vi "MD4Logger.Async.vi"(10 "Parameters":variant, 11 "Process":refnum<class "Process.lvclass">) -> ()   [LabVIEW 2019, in "MD4Logger Engine.lvlib"]
uses:
  MD4Logger Engine.lvlib
  <vilib>/NI/NIVS Inline Async API/_VS Inline Async API/Process/Process.lvclass
  Shared/Compiled.Settings.ctl
  <vilib>/NI/NIVS Inline Async API/_VS Inline Async API/Process/Process.lvclass/Process.ctl
  <vilib>/NI/NIVS Inline Async API/_Data Access Engine/Access Type Classes/Read/Read.lvclass/Read.ctl
  <vilib>/NI/NIVS Inline Async API/_Data Access Engine/Access Type Classes/Write/Write.lvclass/Write.ctl
  <vilib>/NI/NIVS Inline Async API/_Data Access Engine/Data Access Engine/Methods/Read.Data.vi
  <vilib>/NI/NIVS Inline Async API/_Data Access Engine/Data Access Engine/Methods/Write.Data.vi
  <vilib>/NI/NIVS Inline Async API/_VS Inline Async API/Process/Data Member Access/Read Data Access.vi
  <vilib>/NI/NIVS Inline Async API/_VS Inline Async API/Error Handling Process/SubVIs/Error.ConvertArray.vi
  <vilib>/NI/NIVS Inline Async API/_Data Access Engine/Access Type Classes/Read/Read.ProcessData.vi
  <vilib>/NI/NIVS Inline Async API/_Data Access Engine/Access Type Classes/Write/Write.ProcessData.vi
  <vilib>/NI/NIVS Inline Async API/_Data Access Engine/Data Access Engine/Methods/Write.Lookup.vi
  <vilib>/NI/NIVS Inline Async API/_Data Access Engine/Data Access Engine/Methods/Read.Lookup.vi
  <vilib>/NI/NIVS Inline Async API/_Data Access Engine/Data Access Engine/Data Access Engine.lvclass
  Shared/MD4Logger Shared.lvlib
  <vilib>/NI VeriStand/Custom Device Tools/Custom Device Utility Library/Custom Device Utility Library.lvlib
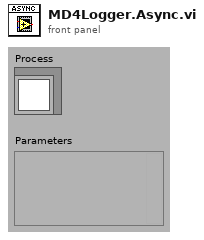
[diagram p1: front panel]
types:
  T1 = typedef "MD4Logger Shared.lvlib/Compiled.Settings.ctl" = cluster{"Name":string, "Folder Path":path, "Channnel Names":cluster{"Name":string, "Unit":string}[]}
  T2 = cluster{"Comment":string, "Time Source":string, "Author":string, "Department":string, "Project":string, "Subject":string}
  T3 = cluster{"History":string, "ID":string, "Vendor":string, "Version":string}
  T4 = typedef "Data Access Engine.lvlib/Data Access Engine.lvclass/Write.DVR.ctl" = refnum<data-value>
  T5 = typedef "Data Access Engine.lvlib/Data Access Engine.lvclass/Read.DVR.ctl" = refnum<data-value>
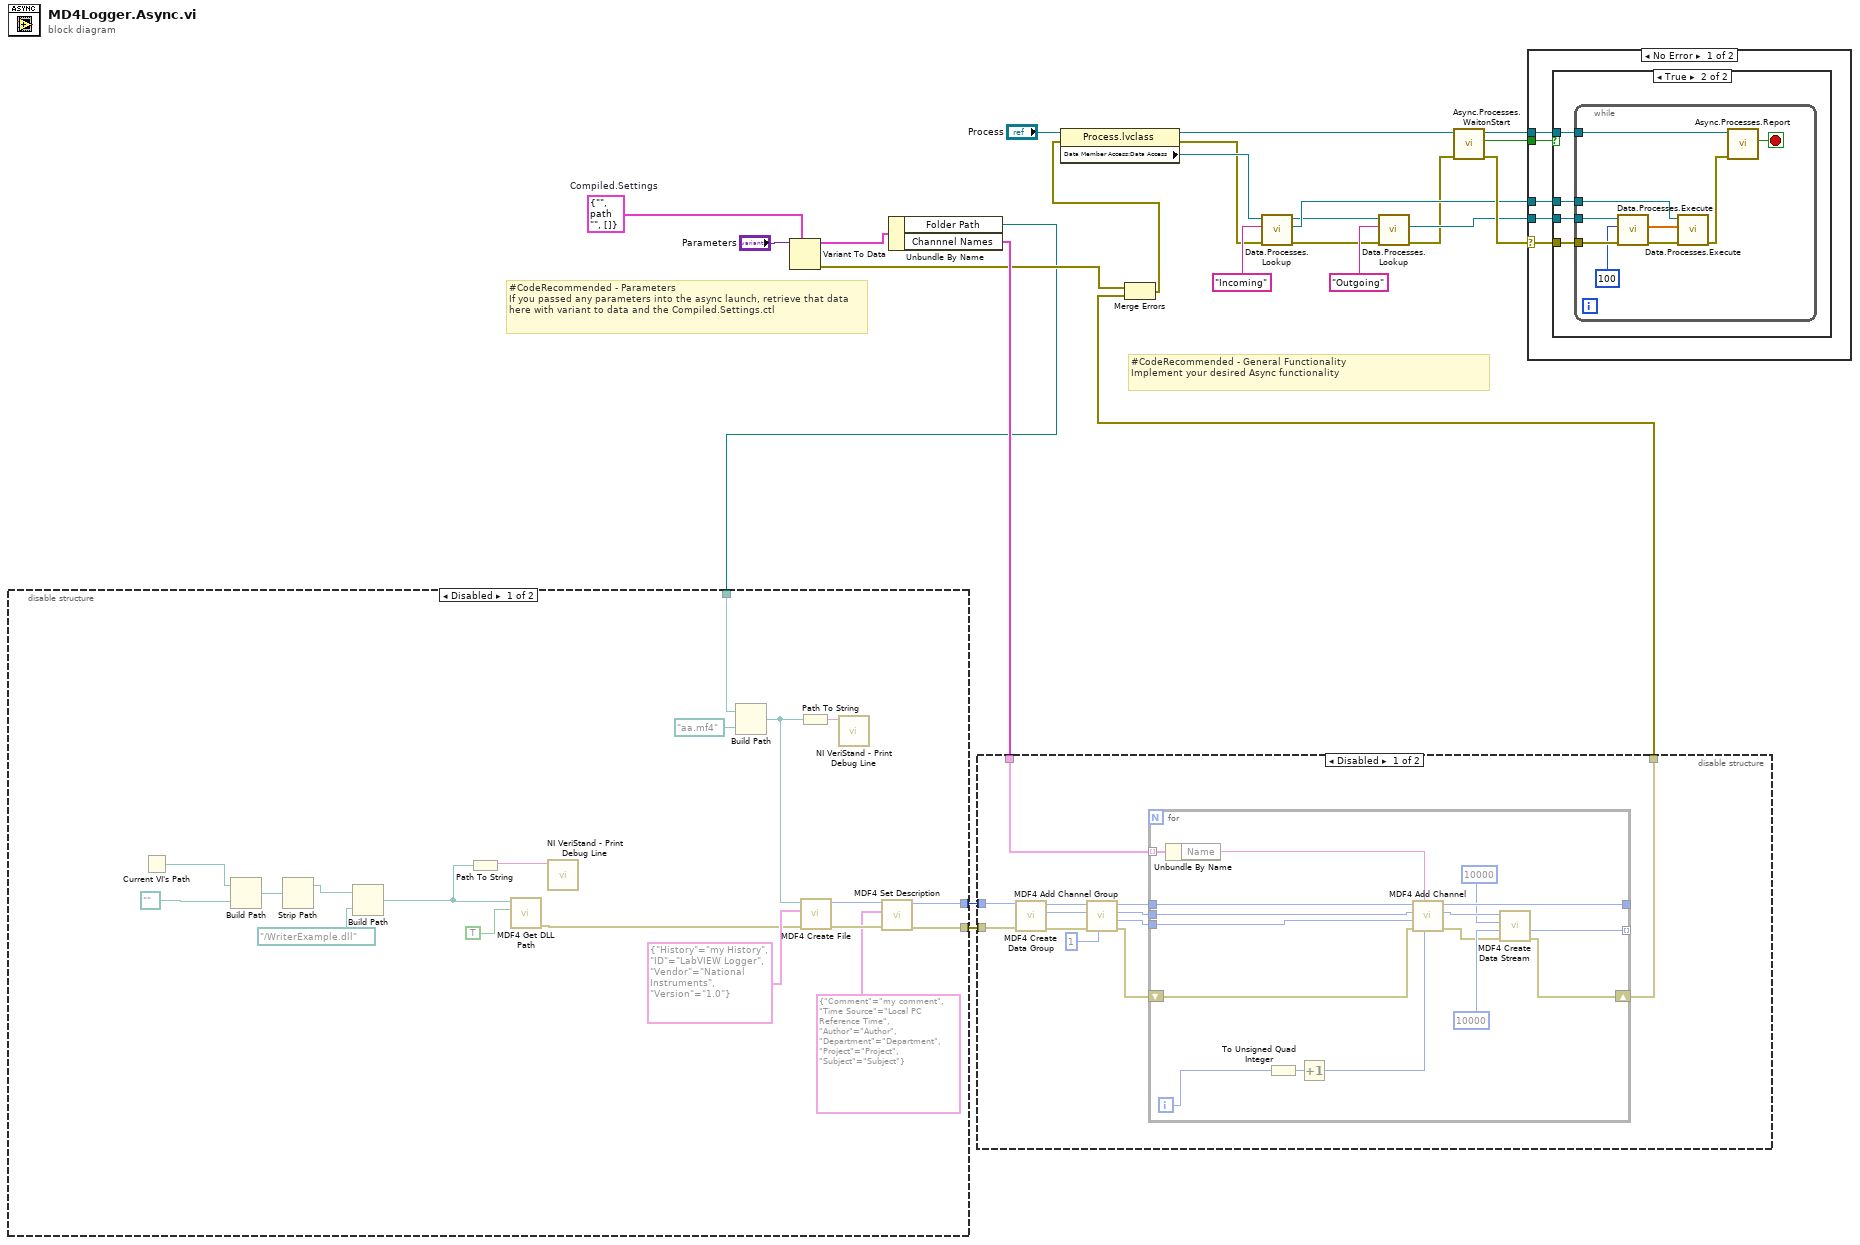
[diagram p0: block diagram]
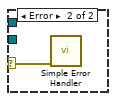
[diagram p5: hidden frame]
diagram:
  w9 = T1 {"Name"="", "Folder Path"=path "", "Channnel Names"=[]}  # Compiled.Settings
  # "#CodeRecommended - General Functionality\nImplement your desired Async functionality"
  # "#CodeRecommended - Parameters\nIf you passed any parameters into the async launch, retrieve that data here with variant to data and the Compiled.Settings.ctl"
  n1 = Variant To Data(type=w9, Variant="Parameters") -> (data=w8:T1, error out=w6:errorcluster)  [unwired: 1 in]
  n2 = Unbundle By Name(w8) -> ("Folder Path"=w1:path, "Channnel Names"=w7:cluster{"Name":string, "Unit":string}[])
  n3 = disable-structure shown="Disabled" {
    disable-tunnel: [w35 _] -> w3
    disable-tunnel: [w34 _] -> w2
    disable-tunnel: w1 -> [w26 _]
    frame Disabled {
      n4 = Current VI's Path() -> (path=w42:path)
      n5 = Build Path(base path=w42, name or relative path=path "..") -> (appended path=w40:path)
      n6 = Strip Path(path=w40) -> (stripped path=w39:path)  [unwired: 1 out]
      n7 = Build Path(base path=w39, name or relative path=path "../WriterExample.dll") -> (appended path=w29:path)
      n8 = Path To String(path=w29) -> (string=w43:string)
      n9 = call "MDF4 Get DLL Path.vi"("Init"=TRUE, "DLL Path"=w29) -> ("error out"=w30:errorcluster)  [unwired: 8 in, 1 out]
      n10 = call <vilib>:"NI VeriStand - Print Debug Line.vi"("Message"=w43) -> ()  [unwired: 10 in, 1 out]
      n11 = Build Path(base path=w26, name or relative path=path "aa.mf4") -> (appended path=w25:path)
      n12 = Path To String(path=w25) -> (string=w28:string)
      n13 = call "MDF4 Create File.vi"("Error In"=w30, "History"=T3 {"History"="my History", "ID"="LabVIEW Logger", "Vendor"="National Instruments", "Version"="1.0"}, "MDF4 File Path"=w25) -> ("Error Out"=w36:errorcluster, "MDF4 File Reference out"=w37:i64)  [unwired: 6 in]
      n14 = call <vilib>:"NI VeriStand - Print Debug Line.vi"("Message"=w28) -> ()  [unwired: 10 in, 1 out]
      n15 = call "MDF4 Set Description.vi"("Error In"=w36, "Comment"=T2 {"Comment"="my comment", "Time Source"="Local PC Reference Time", "Author"="Author", "Department"="Department", "Project"="Project", "Subject"="Subject"}, "MDF4 File Reference in"=w37) -> ("Error Out"=w35:errorcluster, "MDF4 File Reference out"=w34:i64)  [unwired: 7 in]
    }
    frame Enabled {
    }
  }
  n16 = disable-structure shown="Disabled" {
    disable-tunnel: w7 -> [w55 _]
    disable-tunnel: [w54 w72] -> w5
    disable-tunnel: w3 -> [w53 w72]
    disable-tunnel: w2 -> [w52 _]
    frame Disabled {
      n17 = call "MDF4 Create Data Group.vi"("Error In"=w53, "MDF4 File Reference in"=w52) -> ("Error Out"=w51:errorcluster, "Data Group Reference out"=w50:i64, "MDF4 File Reference out"=w49:i64)  [unwired: 7 in]
      n18 = call "MDF4 Add Channel Group.vi"("Record ID"=u64 1, "Error In"=w51, "Data Group Reference in"=w50, "MDF4 File Reference in"=w49) -> ("Error Out"=w48:errorcluster, "Channel Group Reference out"=w45:i64, "Data Group Reference out"=w46:i64, "MDF4 File Reference out"=w47:i64)  [unwired: 4 in]
      n19 = for {
        tunnel: [w71] -> _ mode=indexing
        tunnel: [w70] -> _
        shift-right: [w69] -> w54
        shift-left: w48 -> [w62]
        tunnel: w47 -> [w61]
        tunnel: w46 -> [w60]
        tunnel: w45 -> [w59]
        tunnel: w55 -> [w57] mode=indexing
        i -> [w63]
        n20 = Unbundle By Name(w57) -> ("Name"=w56:string)
        n21 = To Unsigned Quad Integer(1:w63) -> (0:w68:u64)
        n22 = Increment(x=w68) -> (x+1=w58:u64)
        n23 = call "MDF4 Add Channel.vi"("Channel ID"=w58, "Channel Name"=w56, "Error In"=w62, "Channel Group Reference in"=w59, "Data Group Reference in"=w60, "MDF4 File Reference in"=w61) -> ("Error Out"=w64:errorcluster, "Data Group Reference out"=w67:i64, "MDF4 File Reference out"=w70:i64)  [unwired: 3 in]
        n24 = call "MDF4 Create Data Stream.vi"("Error In"=w64, "Number of Samples per Read"=u32 10000, "Iterations"=u32 10000, "Data Group Reference in"=w67) -> ("Error Out"=w69:errorcluster, "Stream Reference out"=w71:i64)  [unwired: 5 in, 1 out]
      }
    }
    frame Enabled {
    }
  }
  n25 = Merge Errors(w6, w5) -> (w4:errorcluster)
  n26 = property class="Process.lvclass"(reference="Process", error in=w4) -> (reference out=w13:refnum<class "Process.lvclass">, error out=w11:errorcluster, "Data Member Access:Data Access"=w12:refnum<class "Data Access Engine.lvclass">)
  n27 = call-poly <vilib>:"Data.Processes.Lookup.vi"("error in (no error)"=w11, "Name"="Incoming", "Data Access API in"=w12) -> ("error out"=w18:errorcluster, "Ref"=w17:T4, "Data Access API out"=w16:refnum<class "Data Access Engine.lvclass">)  [unwired: 5 in, 1 out]
  n28 = call-poly <vilib>:"Data.Processes.Lookup.vi"("error in (no error)"=w18, "Name"="Outgoing", "Data Access API in"=w16) -> ("error out"=w15:errorcluster, "Ref"=w20:T5)  [unwired: 5 in, 2 out]
  n29 = call <vilib>:"Async.Processes.WaitonStart.vi"("error in (no error)"=w15, "Process"=w13) -> ("error out"=w22:errorcluster, "Execute"=w24:bool, "Process out"=w23:refnum<class "Process.lvclass">)  [unwired: 7 in]
  n30 = case shown="No Error" w22 {
    selector: w22 -> [w73 w91]
    tunnel: w24 -> [w77 _]
    tunnel: w23 -> [w76 _]
    tunnel: w17 -> [w75 _]
    tunnel: w20 -> [w74 _]
    frame No Error {
      n31 = case shown="True" w77 {
        tunnel: w73 -> [_ w78]
        tunnel: w76 -> [_ w79]
        tunnel: w74 -> [_ w81]
        tunnel: w75 -> [_ w80]
        frame False {
        }
        frame True {
          n32 = while {
            tunnel: w78 -> [w86]
            tunnel: w79 -> [w90]
            tunnel: w81 -> [w88]
            tunnel: w80 -> [w87]
            stop <- w89 stop-if-true
            n33 = call-poly <vilib>:"Data.Processes.Execute.vi"("error in (no error)"=w86, "timeout ms"=100, "Ref"=w88) -> ("error out"=w84:errorcluster, "Values"=w83:dbl[])  [unwired: 6 in, 1 out]
            n34 = call-poly <vilib>:"Data.Processes.Execute.vi"("error in (no error)"=w84, "Values"=w83, "Ref"=w87) -> ("error out"=w82:errorcluster)  [unwired: 8 in]
            n35 = call <vilib>:"Async.Processes.Report.vi"("Error"=w82, "Process in"=w90) -> ("Stop"=w89:bool)  [unwired: 8 in, 1 out]
          }
        }
      }
    }
    frame Error {
      n36 = call <vilib>:"Simple Error Handler.vi"("error in (no error)"=w91) -> ()  [unwired: 4 in, 5 out]
    }
  }
